vi "Attenuation Cutoff UI.vi"() -> ()   [LabVIEW 2010]
panel:
  in  "Number of \"Open Session\" Retry Attempts (3)":i32=3
  in  "MICS Power Setting (0x16)":u8=22 format="%02x"
  in  "245TX_Power (6)":i8=6
  in  "MICS inputs":T1={"address"="COM5", "chan"=2, "ID"=4412} {"ID" format="%04x"; "chan" min=1 max=10 step=1}
  in  "Samples":i32=10
  in  "Attenuation Range":cluster{"Min":dbl, "Max":dbl, "Increment":dbl}={"Min"=10.0, "Max"=20.0, "Increment"=1.0}
  out "error out":errorcluster
  out "Percent Successful vs. Attenuation":cluster{dbl, dbl}[](graph)
  in  "stop":bool
  in  "error in (no error)":errorcluster
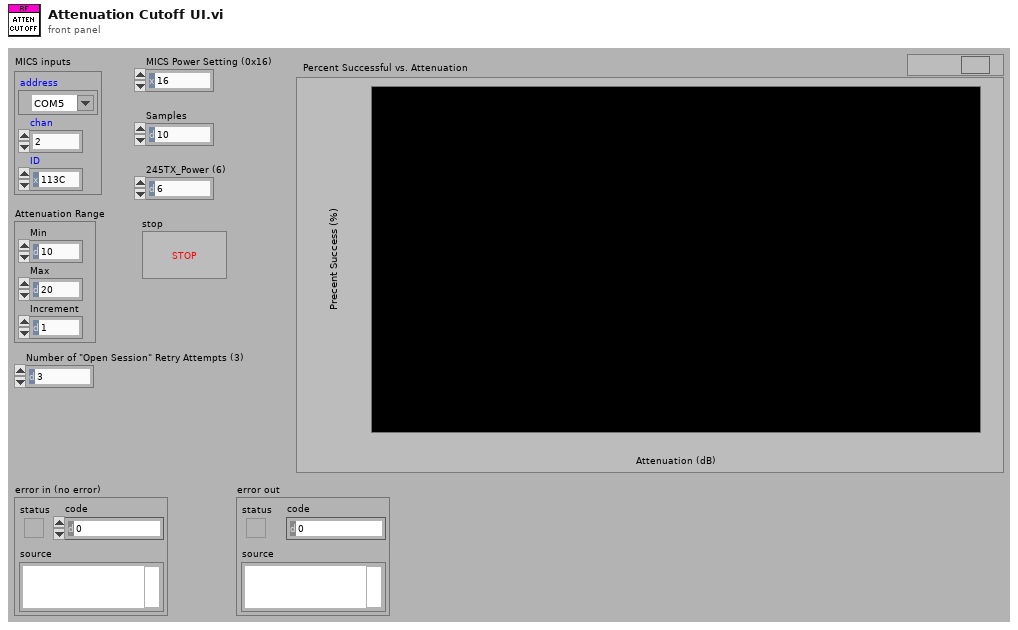
[diagram p1: front panel]
types:
  T1 = cluster{"address":refnum<visa-resource-name>, "chan":u16, "ID":u32}
  T2 = cluster{"ConfigFlags":u8, "ImplantID":u32, "CompanyID":u8, "Normal_Comm":cluster{"RF_Channel":u8, "UserData":u8, "TX_Mod":u8, "RX_Mod":u8, "RX_BlockSize":u8, "BlockPerPack":u8, "TX_BlockSize":u8}, "Emerg_Comm":cluster{"RF_Channel":u8, "UserData":u8, "TX_Mod":u8, "RX_Mod":u8, "TX_BlockSize":u8, "BlockPerPack":u8, "RX_BlockSize":u8}, "ImplantRev":u8, "245TX_PowerCal":i8, "245TX_Power":i8, "CCA_RSSI_Thresholds":cluster{"ch0":u16, "ch1":u16, "ch2":u16, "ch3":u16, "ch4":u16, "ch5":u16, "ch6":u16, "ch7":u16, "ch8":u16, "ch9":u16}}
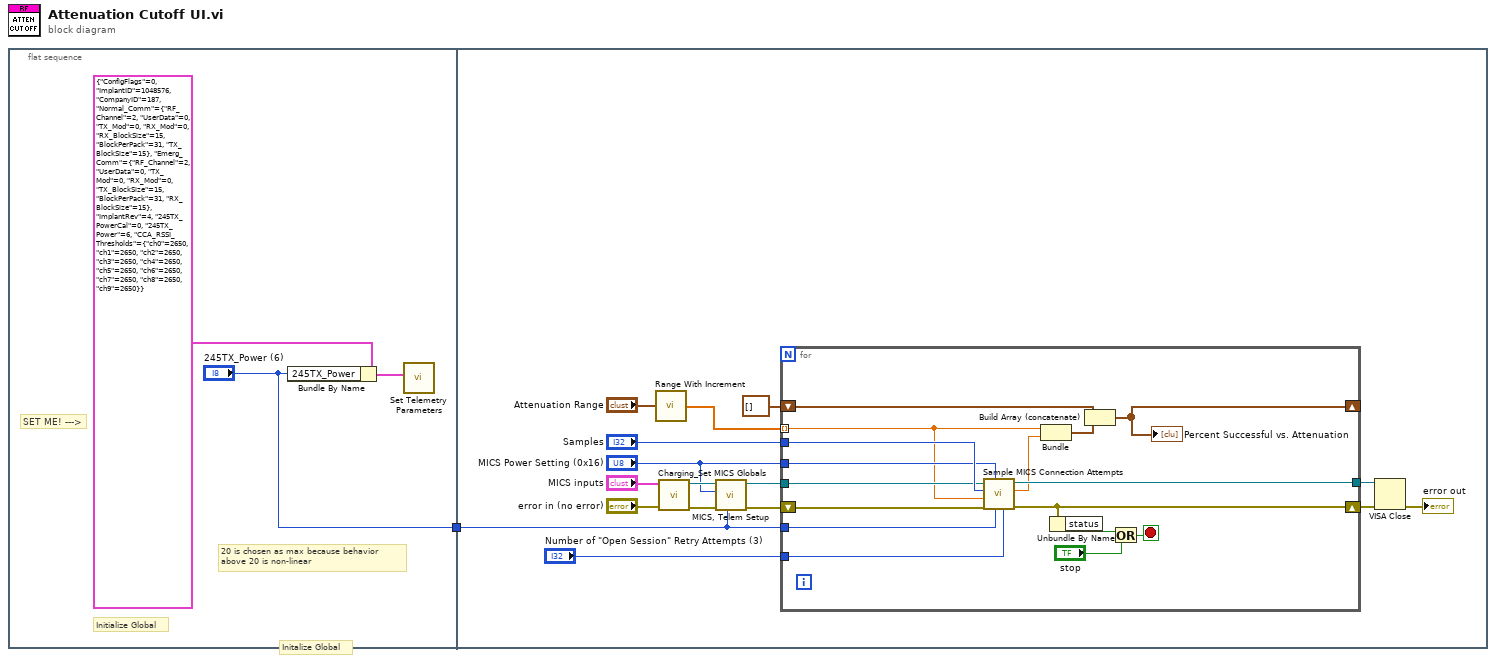
[diagram p0: block diagram]
diagram:
  n1 = flat-sequence {
    tunnel: ["245TX_Power (6)"] -> w1
    tunnel: w1 -> [w5]
    frame #0 {
      # "20 is chosen as max because behavior\nabove 20 is non-linear"
      # "Initialize Global"
      # "SET ME! --->"
      # "Initalize Global"
      n2 = Bundle By Name(cluster=T2 {"ConfigFlags"=0, "ImplantID"=1048576, "CompanyID"=187, "Normal_Comm"={"RF_Channel"=2, "UserData"=0, "TX_Mod"=0, "RX_Mod"=0, "RX_BlockSize"=15, "BlockPerPack"=31, "TX_BlockSize"=15}, "Emerg_Comm"={"RF_Channel"=2, "UserData"=0, "TX_Mod"=0, "RX_Mod"=0, "TX_BlockSize"=15, "BlockPerPack"=31, "RX_BlockSize"=15}, "ImplantRev"=4, "245TX_PowerCal"=0, "245TX_Power"=6, "CCA_RSSI_Thresholds"={"ch0"=2650, "ch1"=2650, "ch2"=2650, "ch3"=2650, "ch4"=2650, "ch5"=2650, "ch6"=2650, "ch7"=2650, "ch8"=2650, "ch9"=2650}} ("MICS_Config_In"), "245TX_Power"="245TX_Power (6)") -> (w3:T2)
      n3 = call "Set Telemetry Parameters.vi"("MICS_Config_In"=w3) -> ()  [unwired: 11 in]
    }
    frame #1 {
      n4 = call "Range With Increment.vi"("Range"="Attenuation Range") -> ("Output Array"=w8:dbl[])
      n5 = call "Charging_Set MICS Globals.vi"("error in"="error in (no error)", "MICS inputs"="MICS inputs") -> ("error out"=w11:errorcluster, "address"=w13:refnum<visa-resource-name>)  [unwired: 4 in]
      n6 = call "MICS, Telem Setup.vi"("2.45 GHz Wake-Up Power (6)"=w5, "error in"=w11, "400 MHz MICS Power Setting (0x16)"="MICS Power Setting (0x16)", "VISA resource"=w13) -> ("error out"=w10:errorcluster, "VISA resource dup"=w9:refnum<visa-resource-name>)  [unwired: 6 in]
      n7 = for {
        shift-right: [w34] -> _
        shift-left: cluster{dbl, dbl}[] [] ("XY Graph") -> [w36]
        tunnel: [w33] -> w19
        tunnel: w8 -> [w23] mode=indexing
        tunnel: "Samples" -> [w27]
        tunnel: w9 -> [w25]
        shift-right: [w32] -> w18
        shift-left: w10 -> [w26]
        tunnel: "MICS Power Setting (0x16)" -> [w24]
        tunnel: w5 -> [w22]
        tunnel: "Number of \"Open Session\" Retry Attempts (3)" -> [w21]
        stop <- w30 stop-if-true
        n8 = call "Sample MICS Connection Attempts.vi"("Number of \"Open Session\" Retry Attempts (3)"=w21, "2.45 GHz Wake-Up Power"=w22, "400 MHz MICS Power Setting"=w24, "error in"=w26, "Attenuation dB"=w23, "Samples (1)"=w27, "MICS Resource Name"=w25) -> ("error out"=w32:errorcluster, "Percent Successful"=w28:dbl, "MICS Resource Name out"=w33:refnum<visa-resource-name>)  [unwired: 1 in, 1 out]
        n9 = Bundle(w23, "Percent Successful"=w28) -> (w35:cluster{dbl, "Percent Successful":dbl})  [unwired: 1 in]
        n10 = Unbundle By Name(w32) -> ("status"=w31:bool)
        n11 = Build Array (concatenate)(w36, w35) -> (w34:cluster{dbl, "Percent Successful":dbl}[])
        "Percent Successful vs. Attenuation" <- w34
        n12 = Or(x=w31, y="stop") -> (x .or. y?=w30:bool)
      }
      n13 = VISA Close(VISA resource name=w19, error in (no error)=w18) -> (error out=→"error out":errorcluster)
    }
  }
